vi "Lockin-4461_Multiple Inputs and Outputs_KH_functional_global_waveform_3.vi"(8 "stop":bool) -> ()   [LabVIEW 2013]
uses:
  <vilib>/Analysis/4window.llb/windowTd.ctl
  <vilib>/DAQmx/write.llb/DAQmx Write (Analog 1D Wfm NChan NSamp).vi
  <vilib>/Analysis/baseanly.llb/Mean (DBL).vi
  <vilib>/Analysis/2dsp.llb/Decimate (single shot).vi
  <vilib>/Analysis/2dsp.llb/Decimate (single shot, DBL).vi
  DAQ-Lockin-SubVI/Lock-in Globles Multiple Inputs and Outputs used with FGV.vi
  <vilib>/DAQmx/miscellaneous.llb/DAQmx Fill In Error Info.vi
  <vilib>/Utility/error.llb/Error Cluster From Error Code.vi
  <vilib>/measure/madcrms.llb/Basic Averaged DC-RMS for N Chan.vi
  <vilib>/measure/macond.llb/IIR Filter for N Chan.vi
  <vilib>/measure/maspectr.llb/FFT Power Spectrum and PSD for N Chan.vi
  <vilib>/Analysis/NI_AALBase.lvlib
  <vilib>/measure/NI_MAPro.lvlib
  <vilib>/measure/NI_MABase.lvlib
  <vilib>/Analysis/NI_AALPro.lvlib
panel:
  in  "order":i32=2
  in  "TC (s)":dbl
  out "filter fC (Hz)":dbl
  in  "Input Signals":i16(slide)=2 scale=1.0..20.0
  out "phase log":dbl[](array[numeric])=[0.0, 0.0, 0.0, 0.0, 0.0, 6.661338147750939e-16, 0.0, 1.9984014443252818e-15]
  in  "Tab Control 2":T1(tab)=enum."Lock-in Settings"
  in  "Auto control  max AI rate/ AI block size":bool=TRUE
  in  "AI Buffer Size (S)":i32=10
  in  "AI Block Size":i32=1000
  in  "AI Configuration":T2(array[cluster])=[{"AI.Coupling"=10050, "AI.Max"=10.0, "AI.Min"=-10.0, "Input physical channels"="PXI1Slot2/ai0:1"}, {"AI.Coupling"=10050, "AI.Max"=10.0, "AI.Min"=-10.0, "Input physical channels"="PXI1Slot3/ai0:1"}, {"AI.Coupling"=10050, "AI.Max"=10.0, "AI.Min"=-10.0, "Input physical channels"="PXI1Slot5/ai0:1"}, {"AI.Coupling"=10050, "AI.Max"=10.0, "AI.Min"=-10.0, "Input physical channels"="PXI1Slot6/ai0:1"}] {"AI.Coupling" items=["AC"=10045, "DC"=10050, "GND"=10066]}
  in  "AO Configuration":T3(array[cluster])=[{"Output physical channels"="PXI1Slot2/ao0:1", "AO. Max"=0.1, "AO.Min"=-0.1}, {"Output physical channels"="PXI1Slot3/ao0:1", "AO. Max"=0.25, "AO.Min"=-0.25}, {"Output physical channels"="PXI1Slot5/ao0:1", "AO. Max"=0.1, "AO.Min"=-0.1}, {"Output physical channels"="PXI1Slot6/ao0:1", "AO. Max"=0.1, "AO.Min"=-0.1}]
  in  "OSC Configuration":T4(array[cluster])=[[{"Signal Type"=enum."Sine Wave", "DC"=0.0, "Amplitude"=0.01, "frequency"=13.0, "Phase"=0.0}, {"Signal Type"=enum."Sine Wave", "DC"=0.0, "Amplitude"=0.0, "frequency"=13.0, "Phase"=0.0}], [{"Signal Type"=enum."Sine Wave", "DC"=0.0, "Amplitude"=0.0, "frequency"=13.0, "Phase"=0.0}, {"Signal Type"=enum."Sine Wave", "DC"=0.0, "Amplitude"=0.0, "frequency"=13.0, "Phase"=0.0}], [{"Signal Type"=enum."Sine Wave", "DC"=0.0, "Amplitude"=0.0, "frequency"=13.0, "Phase"=0.0}, {"Signal Type"=enum."Sine Wave", "DC"=0.0, "Amplitude"=0.0, "frequency"=13.0, "Phase"=0.0}], [{"Signal Type"=enum."Sine Wave", "DC"=0.0, "Amplitude"=0.0, "frequency"=13.0, "Phase"=0.0}, {"Signal Type"=enum."Sine Wave", "DC"=0.0, "Amplitude"=0.0, "frequency"=13.0, "Phase"=0.0}]] {"frequency" step=0.001 format="%.3p"; "Amplitude" format="%0.2p"; "DC" min=-0.99 max=0.99 format="%.2p"}
  in  "Phase&Tc":T5(array[cluster])=[{"Phase"=0.0, "Time constant"=0.5, "Set Tc"=FALSE, "Autophase"=FALSE, "Order"=0.0}, {"Phase"=0.0, "Time constant"=0.5, "Set Tc"=FALSE, "Autophase"=FALSE, "Order"=0.0}, {"Phase"=0.0, "Time constant"=0.5, "Set Tc"=FALSE, "Autophase"=FALSE, "Order"=0.0}, {"Phase"=0.0, "Time constant"=0.5, "Set Tc"=FALSE, "Autophase"=FALSE, "Order"=0.0}, {"Phase"=0.0, "Time constant"=0.5, "Set Tc"=FALSE, "Autophase"=FALSE, "Order"=0.0}, {"Phase"=0.0, "Time constant"=0.5, "Set Tc"=FALSE, "Autophase"=FALSE, "Order"=0.0}, {"Phase"=0.0, "Time constant"=0.5, "Set Tc"=FALSE, "Autophase"=FALSE, "Order"=0.0}, {"Phase"=0.0, "Time constant"=0.5, "Set Tc"=FALSE, "Autophase"=FALSE, "Order"=0.0}] {"Phase" min=0.0 max=360.0 scale=0.0..360.0}
  in  "Gain":dbl[](array[numeric])=[50000000.0, 50000000.0, 1.0, 1.0, 1.0, 1.0, 1.0, 1.0]
  in  "frequency":dbl=13.0
  out "max ai rate":i32=13000
  out "elapsed time":dbl=138.0
  in  "zero offset":bool
  in  "measure offset":bool
  in  "sample clock multiple (x*f)":i32=1000
  out "AI Rate":dbl=13000.0 format="%.2f"
  out "Display 2":string="-423.350804      n"
  out "Display 1":string="-104.244723      n"
  in  "Remote":bool
  in  "Display":u16(ring) items=["X and Y", "R and Theta"]
  out "Backlog":u8(slide) scale=0.0..100.0
  out "Sampling information":cluster{"Fs":dbl, "#s":dbl}[](array[cluster])=[{"Fs"=13000.0, "#s"=1000.0}]
  out "AO Task":refnum<k21>[](array[refnum])
  out "AI task":refnum<k21>[](array[refnum])
  in  "Tab Control":T6(tab)=enum."Input signals"
  out "Display X (or R) A":dbl[](graph)=[-6.767704118237299e-07, 1.3679095941982762e-06, -8.292119972514093e-07, 1.6081112063430916e-06, -6.48302849428553e-07, 3.3000787620994813e-07, 2.1826626593165523e-07, -4.843594448984296e-07, 7.025229913353154e-07, -4.940803961923873e-07, 5.735003337473624e-07, -3.4668515755027405e-07, -2.4248283537339965e-07, -1.8363287469697745e-08, -3.4589425846339534e-07, 4.6284358832454705e-07, -2.6962179655822256e-07, -1.429402751088828e-07, 9.446578651191532e-08, -5.710117984178673e-09, -5.29242574030563e-07, -7.215176081254315e-08, 2.677231693663559e-07, -2.9474346178622007e-07, 1.6859037233620488e-07, -2.782624102402718e-07, -1.9986912438858682e-07, -3.269593679273288e-08, -2.486510407656373e-07, 5.548402109992747e-07, 9.996987486709427e-08, -6.0130416412624e-08, 9.415818662231201e-08, -2.1083634639079388e-07, 4.091053197976716e-07, -1.1752425483839359e-08, -6.151119173511262e-08, 4.276364767795889e-07, 5.672540816315234e-09, 1.9631938693768442e-07, 3.881923939998436e-07, 3.693414665428258e-07, 2.2443312885204412e-07, -1.0424472343376792e-07, -3.281356459413585e-06, 2.853877661113482e-06, -1.6173510513608656e-06, 2.900242509974247e-07, 3.0449767746807755e-07, -9.53094648189971e-07, 1.19768766975668e-06, -1.6300022513090843e-06, 1.2633381081086798e-06, -1.2597657763077924e-06, 1.5181775758183967e-06, -3.2698180448977813e-07, 4.534684182323745e-22, 2.954958383906869e-22, 2.935987294164666e-22, 2.9919274066034985e-22, 2.4866884846013956e-11, 1.571439962444634e-06, 3.5981993954562916e-05, 4.595320866342681e-05, -3.163614064440566e-05, 2.2025345770237146e-05, -1.4783690228833628e-05, 9.027427496250188e-06, -4.373865947312203e-06, 1.2061179513411652e-06, 2.321934449801555e-06, -3.096117951559957e-06, 3.818767600136303e-06, -2.724223846911526e-06, 2.777457898492608e-06, -1.6318104191727555e-06, 8.644446773102741e-07, 5.245164233996108e-07, -9.074912983112755e-07, 1.5809479476204886e-06, -1.191807434600212e-06, 1.1136104668741203e-06, -8.918436045180084e-07, 7.666775683008394e-07, 4.0094363870758105e-07, -5.024016863890059e-07, 6.184199345905923e-07, -4.547811927193765e-07, 8.577352486006216e-07, -3.929716458984687e-07, -9.250952352542821e-08, 1.4464495001439634e-07, 2.987012020098487e-07, -8.395621078021276e-09, -5.946540278253675e-08, 5.015724336232653e-07, -2.2845172399208505e-07, 2.9148694268542234e-07, -3.3585825169289965e-08, 1.5255809451280384e-07, -1.6688588171069325e-07, 2.9208673634758535e-07, 2.1867560915340566e-08, -1.817033331852077e-09, 2.0922044023006386e-07, -2.0089195447457524e-07, -1.6047621413178067e-07, 3.62693951906398e-07, -4.219972565448854e-07, 2.644775088575862e-07, 1.6782279517097728e-07, -4.0780410649598406e-07, -1.4202551172988562e-07, 4.1098274242707864e-08, 4.0982393853747056e-07, -1.0954576241181e-08, -2.000666884411931e-07, 3.419460779804609e-07, -5.831329333541703e-07, 1.607889368959098e-07, 4.7485928317065607e-07, -1.0986820397700458e-07, 4.234349182513178e-07, 7.50799000900104e-09, -2.913745535551743e-07, 5.212516629832497e-07, -3.5679666811606247e-07, 7.185358920930657e-07, 2.28551626188166e-07, 2.984900132189184e-07, 5.567614355159372e-07, -2.700163649574881e-08, 4.647757728519345e-09, -7.827331963284188e-09, -3.16290394262067e-07, 2.2708072760302243e-07, 7.739366205819891e-08, -4.86859103219973e-07, 2.473259207485168e-07, -3.41601067670072e-07, 1.6627441476941349e-07, 8.910868327391612e-08, -4.126919161116403e-08, 5.064621322918384e-07, -7.216585649893412e-08, 1.7360798289963554e-07, 1.9894946958931327e-07, -1.029870892195247e-07, 1.479174782511515e-08, -7.761128801091328e-08, -9.710807258322806e-08, 2.244692789108791e-07, -5.009546674149695e-07, 2.4630441386600876e-07, 3.701090240857261e-07, -4.940910423104556e-07, 6.97823655978583e-07, 5.463396637012674e-08, 3.3460509656657584e-07, 1.1628795209397034e-07, -9.983904012316269e-08, 2.1194575699660896e-07, -1.4284598126625291e-07, -1.6581535570295627e-07, 1.9543419229659077e-07, 6.421246147653625e-08, 3.817631543808754e-07, 3.5099411367530134e-07, 9.599061510866204e-08, 5.115460403448378e-07, -3.189544820970916e-07, 2.0371122850583007e-07, 7.139469677112191e-08, -2.6780725397357064e-08, 1.8207931762268008e-07, -3.99163483902508e-08, 3.5667336283414435e-24, 2.977721146793187e-22, 2.9488566597725565e-22, 2.931805455672584e-22, 2.8533874679319433e-11, 4.4171853288673887e-07, 1.1776020155369053e-05, 4.5492863810876877e-05, 2.9323742019926304e-05, -2.1525943992685573e-05, 6.085028499678217e-06, 3.4517457636324723e-06, -7.402821485273008e-06, 8.023515280656284e-06, -5.743846711537538e-06, 3.3274091105157146e-06, -7.62703220096605e-07, -1.0696366449954687e-06, 2.5134804524775262e-06, -2.6343637407641244e-06, 2.5318619928474184e-06, -1.7306766758057638e-06, 1.44992950833644e-06, 1.4483945167047895e-07]
  out "Display Y (or Theta) A":dbl[](graph)=[4.765499299686936e-07, -9.658586916637982e-07, -7.621778309143253e-08, -1.5258147249425879e-07, -2.4990753387284357e-07, 1.3419411932204113e-07, -8.565299692875945e-07, 5.571108791407577e-07, -7.860547079397809e-08, -7.196286228942718e-07, 3.4315278763967647e-07, -6.204384175643328e-07, 1.774316085303007e-07, 1.375503590545208e-07, -9.027207823009459e-07, 4.7108028753992357e-07, -1.4273262355224388e-07, -5.084378639622054e-07, 2.0064639544519283e-07, -6.100241361118937e-07, 3.5508186140312606e-07, 1.6599492404614552e-07, -1.1241242632694126e-06, 3.545737663988187e-07, -1.3680834360003273e-07, -5.671646797482132e-07, 3.003111466009731e-07, -7.790822713575479e-07, 3.293880422749827e-07, 3.28274379240407e-08, -1.0651740914596076e-06, 4.2770794764999845e-07, -5.104224380786051e-07, -2.472151922016114e-07, 1.9800282516829894e-07, -7.284254119168647e-07, 5.863115303219669e-07, -2.81773970579004e-07, -7.156335675351997e-07, 2.3981773570157667e-07, -3.978801443495009e-07, 3.035512690481674e-07, -1.7158995838277135e-07, -4.233508035480193e-07, -8.088850970477616e-07, 6.737027936126898e-07, -1.759072178658265e-07, -6.972834404887968e-07, 1.272488135816818e-06, -1.2086621076536852e-06, 4.69525474705048e-07, -4.919175010780031e-08, -3.50864282590232e-07, 6.020350472256037e-07, -9.484640076506137e-07, -6.830224693863262e-08, 1.0170935534147539e-22, -8.29623972830081e-22, -8.014563293027786e-22, -8.094000243152346e-22, 1.3353078985706605e-11, 1.6373548472325611e-07, 1.4866311767580978e-06, -2.707411790797605e-06, 6.830995141435044e-07, -3.8763934216822793e-07, -3.894235373830128e-07, -9.303274404957174e-08, -1.5541472171160917e-07, -1.0548850159824638e-06, 1.301686262269789e-06, -1.9557074574821375e-06, 9.368644690210887e-07, -5.392324932206546e-07, -1.0317815283114626e-06, 9.503284335604831e-07, -1.1138402195810916e-06, -8.612001299094237e-08, 3.392287632745269e-07, -9.880574731396456e-07, 6.176942647460194e-07, -5.670403477561947e-07, -7.529082791811021e-08, 3.797538713075729e-07, -6.875418705429333e-07, 3.774689030428864e-08, 4.010310610815791e-07, -5.552428738314573e-07, 3.8499536868861883e-07, -6.445873434134007e-07, -3.326615731244241e-07, 4.502182873700019e-07, -7.750874192225206e-07, 4.117923202917222e-07, -6.431352998299419e-07, 3.5044644716276235e-07, -1.4225277208615523e-07, -6.876478797176894e-07, 5.399420578514256e-07, -4.5606838526251626e-07, -1.2810883746936567e-07, 7.507205080273586e-07, -1.4012460201934012e-06, 3.6687827494239255e-07, -2.4916075902104696e-07, -6.048091008906423e-07, 6.617540494081048e-07, -1.017139965154715e-06, 6.302573641557335e-07, 4.555496901851896e-07, -1.3339391648309178e-06, 6.715666266662573e-07, -3.8798990954152797e-07, -3.6012440675569084e-07, 5.414910168700109e-07, -1.3243576755919245e-06, 5.902559482413635e-07, -7.542190392147796e-08, -1.0785352133753382e-06, 9.869413956855774e-07, -9.442478036537707e-07, -4.8555902344221593e-08, 5.874045024703844e-07, -1.1585692990263365e-06, 1.3486079750496373e-06, -5.071584526584705e-07, -5.100916917445276e-07, 6.330937674492109e-07, -1.235592399497452e-06, 9.223862720486185e-07, 6.04251856246877e-08, -1.2764854943402043e-06, 8.83547168218078e-07, -9.047288617993288e-07, 2.0116909352114474e-07, 5.358138396845644e-07, -1.3168565866224215e-06, 4.095307061714363e-07, -6.27867381040266e-07, -4.472555022141913e-07, 8.124683056348434e-07, -6.96815296189946e-07, -1.3075261738966236e-07, -2.448175089906454e-07, -3.31091978464826e-07, 4.938406467055916e-07, -1.0121928097926847e-06, 2.6683471402237015e-07, -3.854622779756573e-07, -6.116229848120615e-07, 7.413846592203119e-07, -3.878576789341664e-07, -4.803212369821987e-09, -1.512740254582647e-07, -9.37733298786493e-07, 3.083451264193004e-07, -7.278473080315107e-07, -2.1621978373244913e-07, 1.1649243053043013e-06, -1.5574296555740364e-06, 2.0216029416288657e-07, -1.738290377715283e-08, -8.124252331847678e-07, 8.556517228357048e-07, -1.1895268912765046e-06, -1.6299284686030149e-07, 5.025591222770188e-07, -1.256876728303257e-06, 4.966801881381768e-07, -2.653578297740131e-07, -7.841925208481243e-07, 6.961355949365849e-07, -1.3545884441334733e-06, 1.8978106285789698e-07, -3.1292466455277164e-07, -1.116079741754174e-06, 6.606025379921262e-24, -7.987352443116322e-22, -8.305769155450611e-22, -8.014315043874178e-22, 1.528632786785048e-11, 5.851716352372578e-08, 7.012774926585611e-07, 7.260202605191567e-07, -1.8385722657507987e-06, -7.48491270371179e-07, 1.078630704871155e-06, -5.895807456908318e-07, 1.4658536078852006e-07, 1.0975439156015532e-07, -4.165723785464372e-07, -6.413089995227893e-08, 2.3302809137460278e-07, -4.5082625792713e-08, 1.8812524970362413e-07, 1.2661990176118822e-08, -9.607065782256097e-07, 4.267709983481109e-07, -7.948677906464168e-08, -2.6388811975329723e-07]
  out "Waveform Graph":waveform(dbl)[](graph)
  in  "decimating factor":i32=1
  in  "simulate?":bool
  in  "pt by pt?":bool
  out "Waveform Graph 2":cluster{"f0":dbl, "df":dbl, "magnitude":dbl[]}[](graph)
  in  "window":T7=1 items=["Rectangle"=0, "Hanning"=1, "Hamming"=2, "Blackman-Harris"=3, "Exact Blackman"=4, "Blackman"=5, "Flat Top"=6, "4 Term B-Harris "=7, "7 Term B-Harris"=8, "Low Sidelobe"=9, "Blackman Nuttall"=11, "Triangle"=30, "Bartlett-Hanning"=31, "Bohman"=32, "Parzen"=33, "Welch"=34, "Kaiser"=60, "Dolph-Chebyshev"=61, "Gaussian"=62]
  in  "averaging parameters":T8={"averaging mode"=enum."No averaging", "weighting mode"=enum."Exponential", "number of averages"=10} {"number of averages" min=1}
  in  "dB On (F)":bool
  out "Results (X, Y, R, Theta)":dbl[][](array[numeric])=[[-8.990938951699043e-08, -5.496874633933286e-07, 5.569919260950825e-07, -99.28930194172699], [-1.0424472343376792e-07, -4.233508035480193e-07, 4.3599640506377615e-07, -103.83315475232594], [-8.663279130692378e-08, -2.555950511771059e-07, 2.6987788111636043e-07, -108.72385784210852], [-3.572835649086049e-08, -7.56786271488616e-08, 8.368853006639814e-08, -115.2722910768039], [4.431812686724637e-08, 8.517364090161592e-08, 9.601377751895176e-08, 62.51083208252897], [1.4523643643592666e-07, 1.9896598237318188e-07, 2.4633530930488284e-07, 53.87219602328508]] format="%#_6p"
  out "Measure?":u16[](array[numeric])
  in  "Cluster (unused right now)":T9={"Amplitude"=[0.001, 2e-08, 0.001, 0.001, 0.001, 2e-08], "DC"=[0.001, 2e-08, 0.001, 0.001, 0.001, 2e-08], "phase"=[0.001, 2e-08, 0.001, 0.001, 0.001, 2e-08], "Array"=[]}
  out "offsets":dbl[](array[numeric])
  # "*****Customized for 4461 + 4462 cards; functional globals*****"
  # "Real time Adjustable Values"
  # "WAVEFORM 2"
  # "Configurations"
  # "should this be x multiple\nof the frequency?"
  # "The top array index selects which card you are setting the outputs for,and the second index selects which output chanel on that card.\n\nFor Phase&Tc, you must have an array element initialized for each input signal."
  # "Features:\n1, Any number of input and output channels\n2, Each AO outputs an DC+AC signal, DC for sample biasing and AC for OSC. These values can be adjusted in real time.\n3, Synchronous filtering\n\nInstructions:\n1, Array index of AI configuration and AO configuration refers to task.\n2, Array index in Amplifier Settings, Phase$&Tc control , and gains correlates to channel number.\n3, Each 4461 board can have 2 lock-in channels. Syntax for 2 channles, e.g. PXI1Slot2/ai0:1. If you want to use just one, then PXI1Slot2/ai0.\n4, Parameters (especially DC value for sample biasing) can be remotely controlled by clicking \"local\"and \"remote\" button. In real experiments, put golable values (can be found in Lock-in globles.vi) in your VI to control the lock-in and read out.\n5, choose OSC frequencies to be multiple of \nAI Rate/AI Block SIze to have best performance.\n\n-Guanglei 06/23/2011\n\nUpdate:\n1. Allows any number of lockin amplifiers and AO tasks.\n2. Delete the channels from any AI/AO Configuration elements you do not want to use.\n3. Rows (first index) of the OSC Configuration correspond to different AO tasks, while columns (second index) correspond to AO channels in that task. All channels in a given element of the AO Configuration array will go into a single task.\n4. The same number of output channels must go in each AO task.\n5. Make sure a Phase&Tc element and an Amplifier Settings element is set for each AI channel.\n-Joe 12/3/2013"
  # "signal\n*sine\n*cosine\n*2\n*2\nLP filter\nLP filter"
  # "hide stuff here in this tab"
  # "multiple of frequency??"
  # "this is \"time constant\""
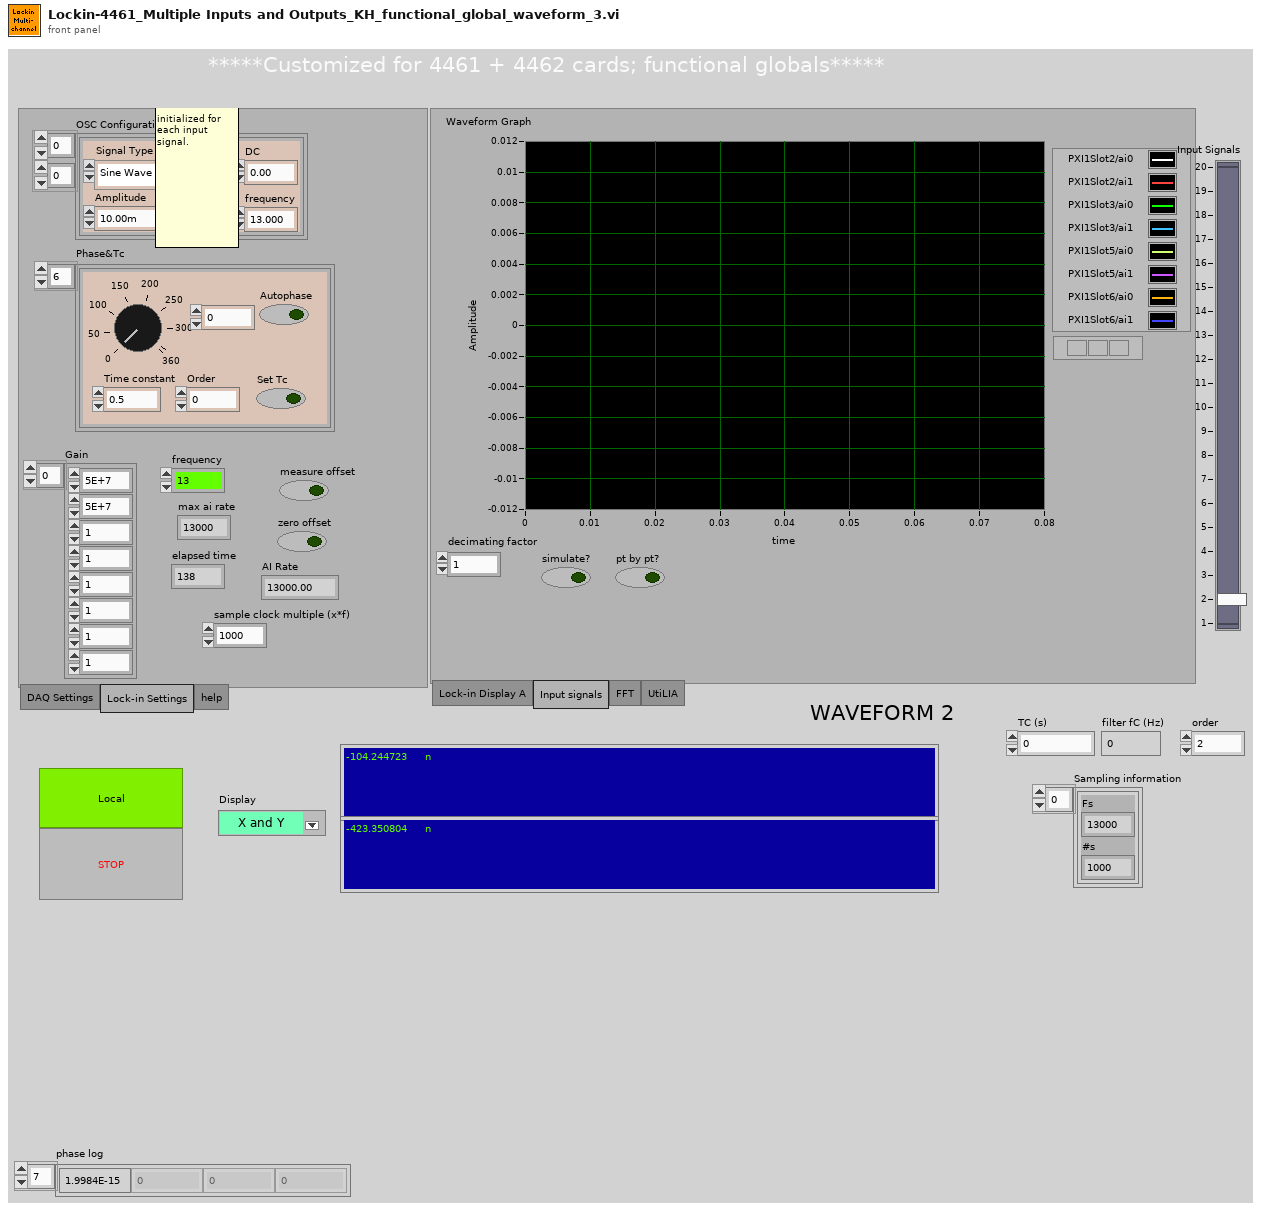
[diagram p1: front panel]
types:
  T1 = enum32{"DAQ Settings", "Lock-in Settings", "help"}
  T2 = cluster{"AI.Coupling":i32, "AI.Max":dbl, "AI.Min":dbl, "Input physical channels":tag}[]
  T3 = cluster{"Output physical channels":tag, "AO. Max":dbl, "AO.Min":dbl}[]
  T4 = cluster{"Signal Type":enum16{"Sine Wave", "Triangle Wave", "Square Wave", "Sawtooth Wave"}, "DC":dbl, "Amplitude":dbl, "frequency":dbl, "Phase":dbl}[][]
  T5 = cluster{"Phase":dbl, "Time constant":dbl, "Set Tc":bool, "Autophase":bool, "Order":dbl}[]
  T6 = enum32{"Lock-in Display A", "Input signals", "FFT", "UtiLIA"}
  T7 = typedef "NI_AALPro.lvlib/windowTd.ctl" = u32
  T8 = cluster{"averaging mode":enum16{"No averaging", "Vector averaging", "RMS averaging", "Peak hold"}, "weighting mode":enum16{"Linear", "Exponential"}, "number of averages":u32}
  T9 = cluster{"Amplitude":dbl[], "DC":dbl[], "phase":dbl[], "Array":enum16{"Sine Wave", "Triangle Wave", "Square Wave", "Sawtooth Wave"}[]}
  T10 = cluster{"Topology":enum16{"Off", "Butterworth", "Chebyshev", "Inverse Chebyshev", "Elliptic", "Bessel"}, "Type":enum16{"Lowpass", "Highpass", "Bandpass", "Bandstop"}, "Order":i32, "Lower Fc":dbl, "Upper Fc":dbl, "PB Ripple":dbl, "SB Attenuation":dbl}
  T11 = cluster{"Signal Type":enum16{"Sine Wave", "Triangle Wave", "Square Wave", "Sawtooth Wave"}, "DC":dbl, "Amplitude":dbl, "frequency":dbl, "Phase":dbl}
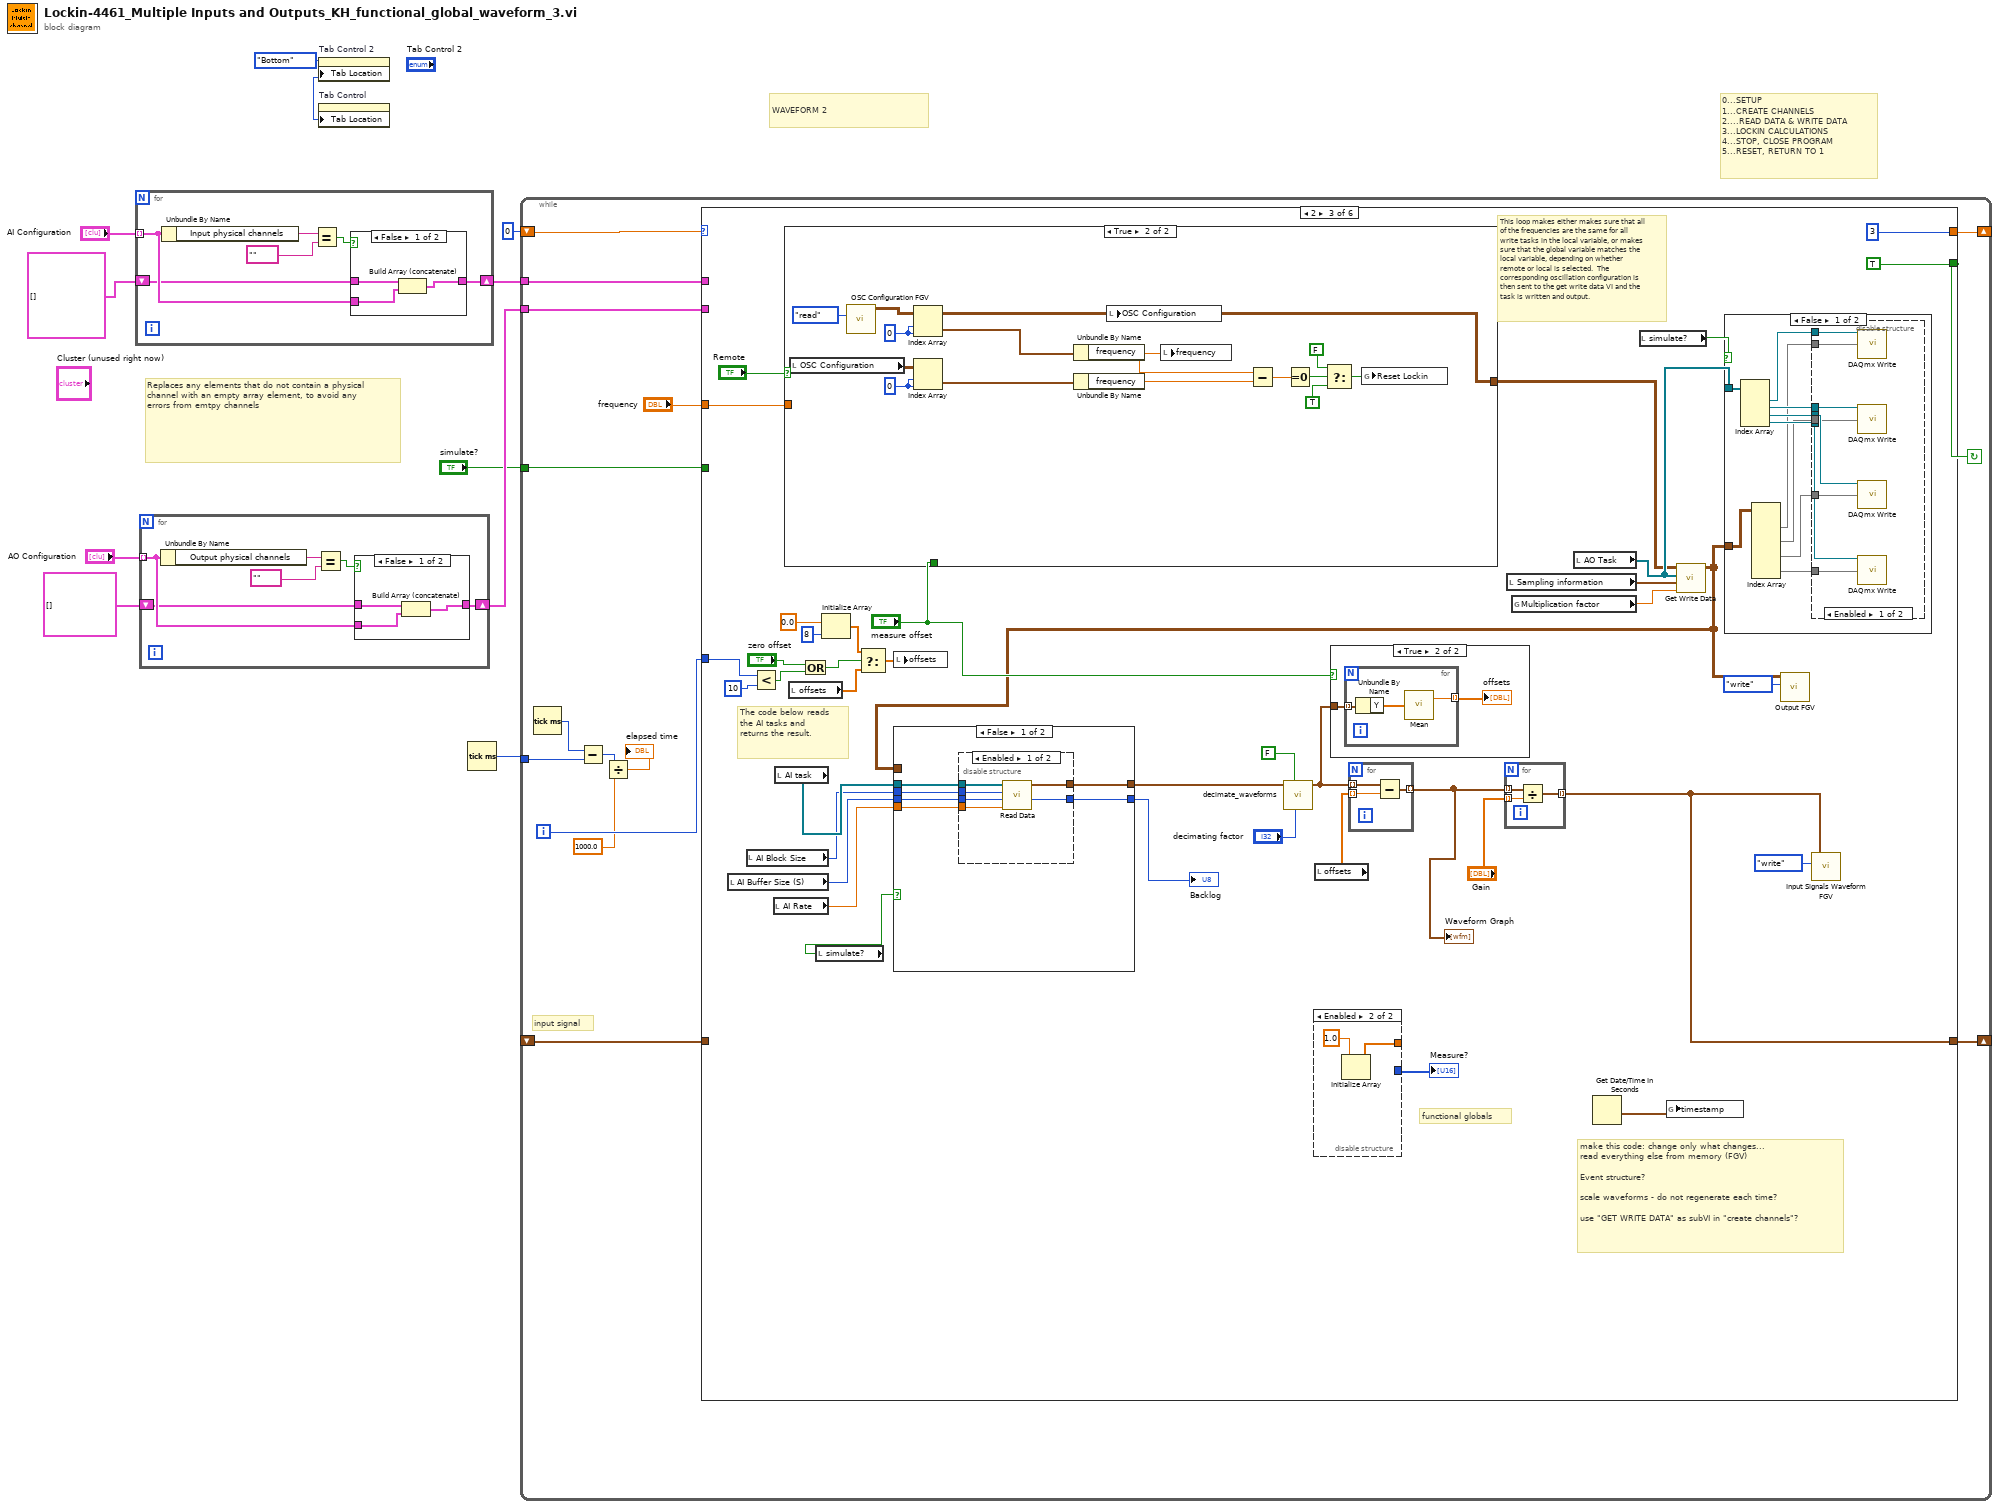
[diagram p0: block diagram]
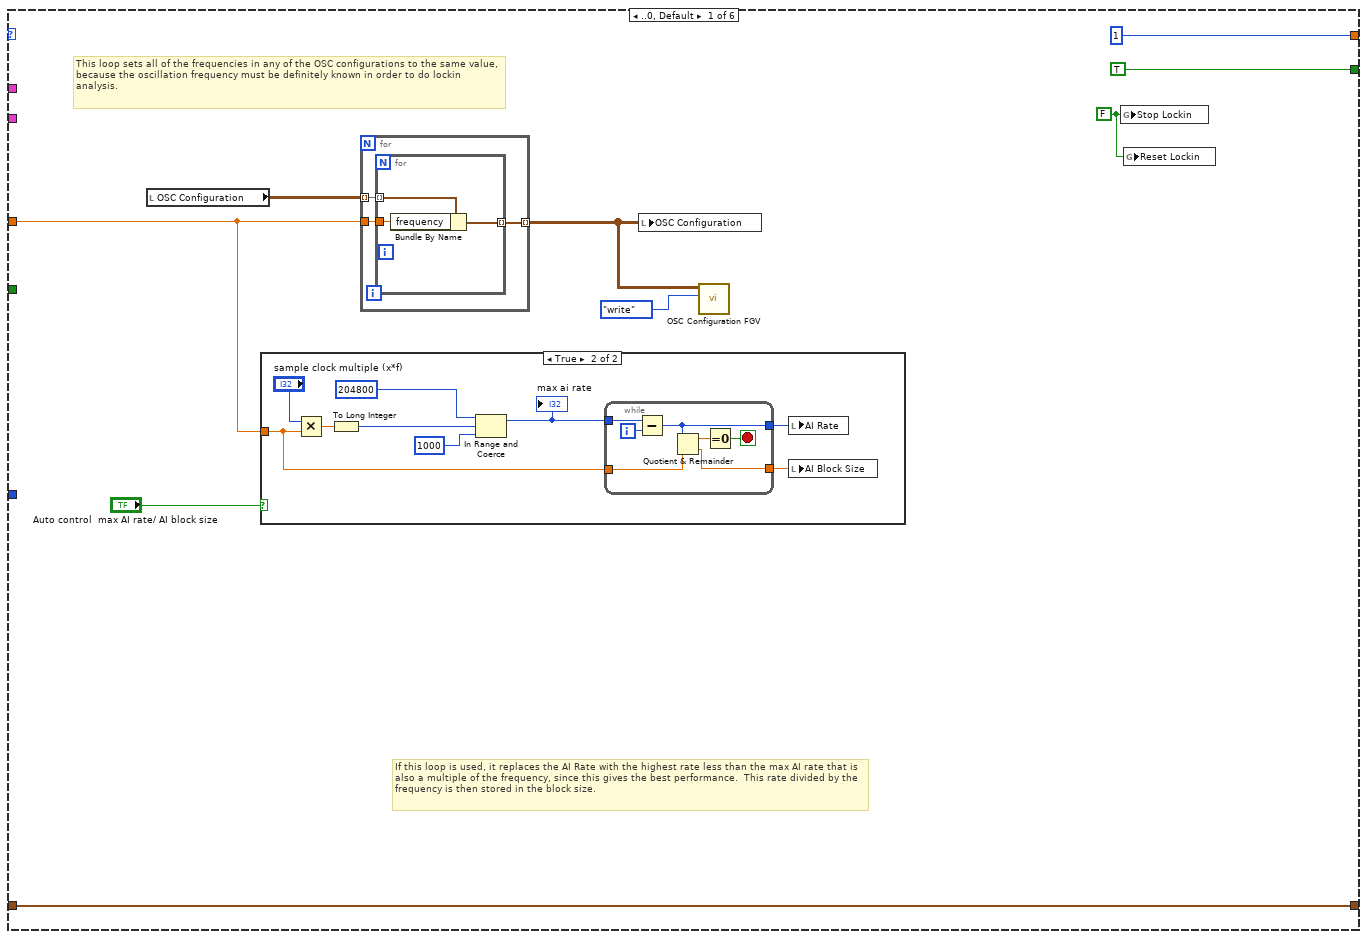
[diagram p4: hidden frame]
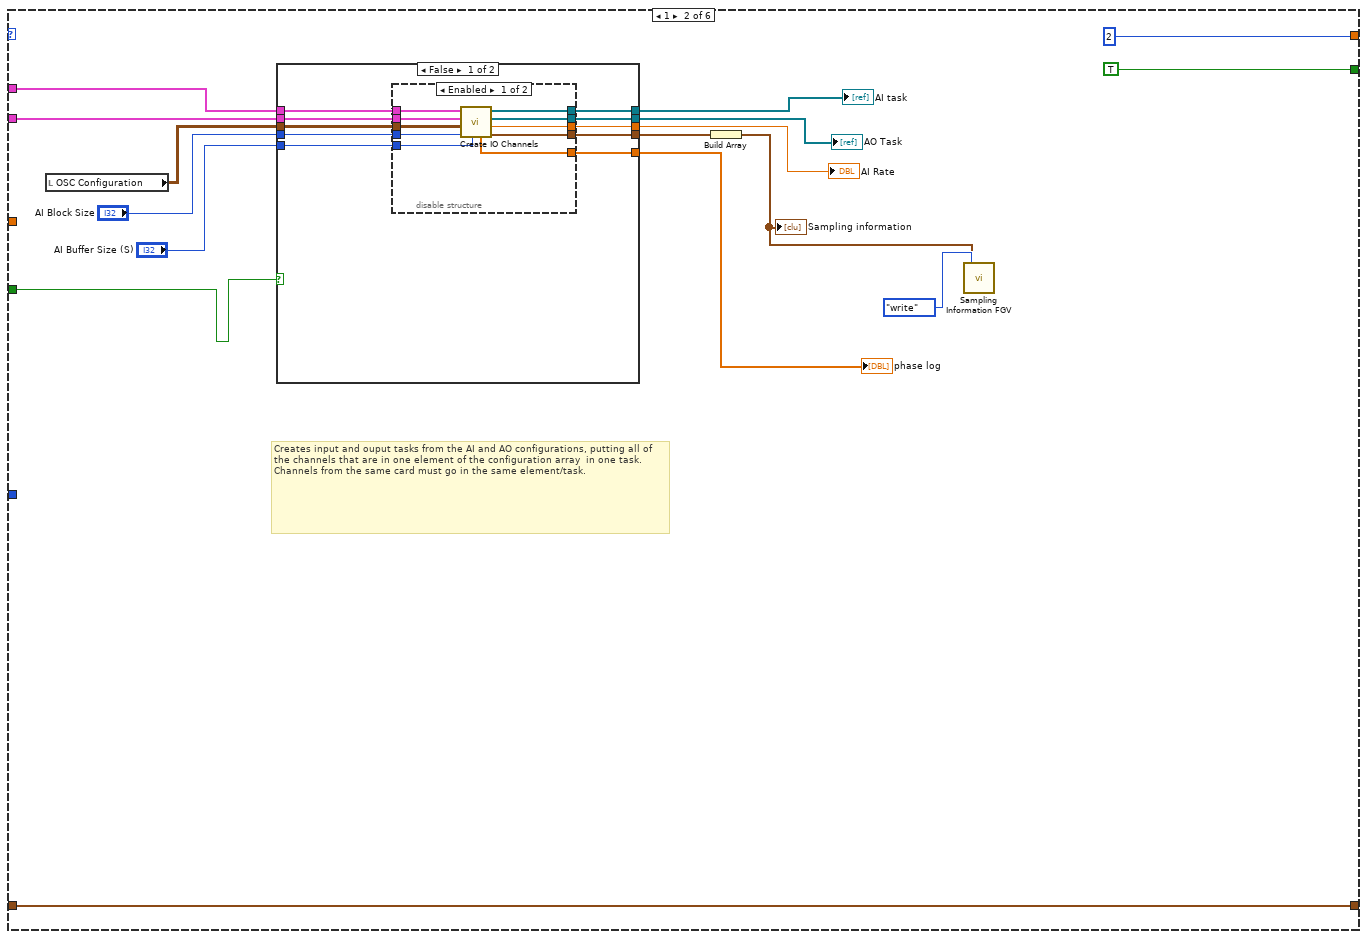
[diagram p6: hidden frame]
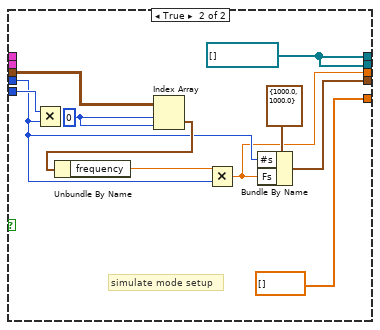
[diagram p8: hidden frame]
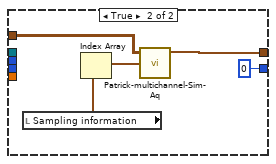
[diagram p12: hidden frame]
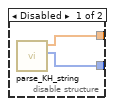
[diagram p14: hidden frame]
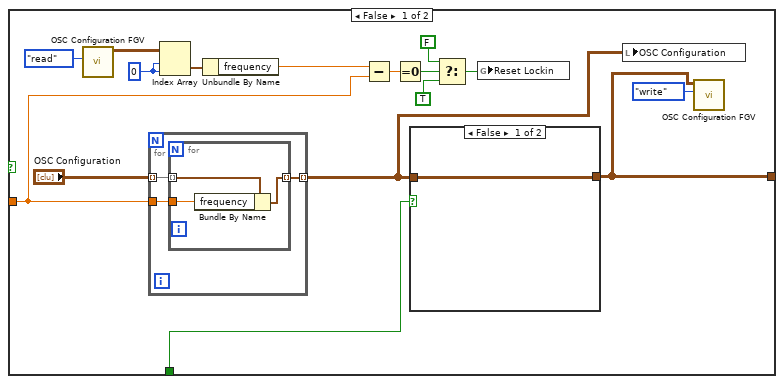
[diagram p15: hidden frame]
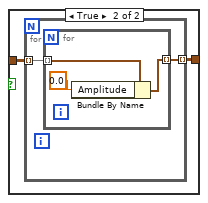
[diagram p16: hidden frame]
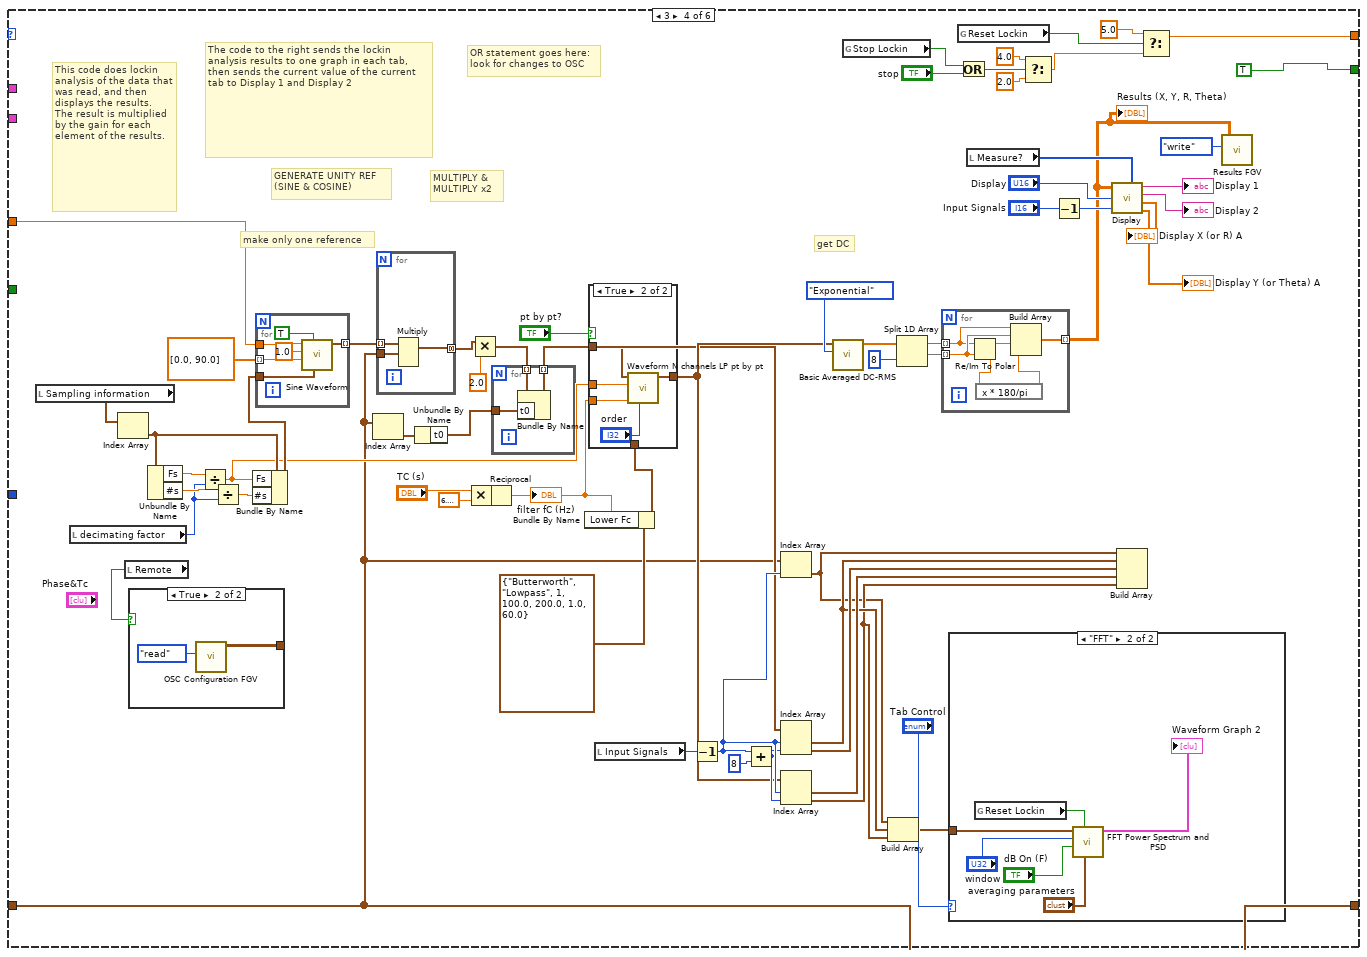
[diagram p17: hidden frame]
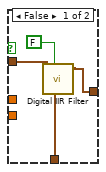
[diagram p18: hidden frame]
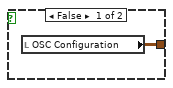
[diagram p20: hidden frame]
diagram:
  w5 = enum32{"Top", "Bottom", "Left", "Right"}."Bottom" ("Tab Location")
  # "0...SETUP\n1...CREATE CHANNELS\n2....READ DATA & WRITE DATA\n3...LOCKIN CALCULATIONS\n4...STOP, CLOSE PROGRAM\n5...RESET, RETURN TO 1"
  # "WAVEFORM 2"
  # "Replaces any elements that do not contain a physical channel with an empty array element, to avoid any errors from emtpy channels"
  n1 = for {
    tunnel: "AI Configuration" -> [w13] mode=indexing
    shift-right: [w11] -> w10
    shift-left: T2 [] ("AI Configuration") -> [w12]
    n2 = Unbundle By Name(w13) -> ("Input physical channels"=w15:tag)
    n3 = Equal?(x=w15, y=tag "" ("Empty physical channels")) -> (x = y?=w16:bool)
    n4 = case shown="False" w16 {
      tunnel: w13 -> [w18 _]
      tunnel: w12 -> [w19 w20]
      tunnel: [w17 w20] -> w11
      frame False {
        n5 = Build Array (concatenate)(w19, w18) -> (w17:T2)
      }
      frame True {
      }
    }
  }
  n6 = for {
    tunnel: "AO Configuration" -> [w23] mode=indexing
    shift-right: [w21] -> w3
    shift-left: T3 [] ("AO Configuration 2") -> [w22]
    n7 = Unbundle By Name(w23) -> ("Output physical channels"=w25:tag)
    n8 = Equal?(x=w25, y=tag "" ("Empty physical channels")) -> (x = y?=w26:bool)
    n9 = case shown="False" w26 {
      tunnel: w23 -> [w28 _]
      tunnel: w22 -> [w29 w30]
      tunnel: [w27 w30] -> w21
      frame False {
        n10 = Build Array (concatenate)(w29, w28) -> (w27:T3)
      }
      frame True {
      }
    }
  }
  n11 = property on="Tab Control 2" class="TabCtl (strict)"("Tab Location"=w5) -> ()  [unwired: 2 in, 2 out]
  n12 = property on="Tab Control" class="TabCtl (strict)"("Tab Location"=w5) -> ()  [unwired: 2 in, 2 out]
  n13 = Tick Count (ms)() -> (millisecond timer value=w2:u32)
  n14 = while {
    shift-right: [w45] -> _
    shift-left: 0 -> [w44]
    tunnel: w10 -> [w43]
    tunnel: w3 -> [w41]
    shift-right: [w40] -> _
    shift-left: _ -> [w39]
    tunnel: w2 -> [w35]
    tunnel: "simulate?" -> [w31]
    i -> [w38]
    stop <- w42 continue-if-true
    # "input signal"
    n15 = Tick Count (ms)() -> (millisecond timer value=w36:u32)
    n16 = Subtract(x=w36, y=w35) -> (x-y=w34:u32)
    n17 = Divide(x=w34, y=1000.0) -> (x/y=→"elapsed time":dbl)
    n18 = case shown="2" w44 {
      selector: w44 -> [_ _ _ _ w358 _]
      tunnel: [1 2 3 w311 w358 0.0 ("f")] -> w45
      tunnel: w43 -> [_ w89 _ _ _ _]
      tunnel: [TRUE TRUE TRUE TRUE FALSE TRUE] -> w42
      tunnel: w41 -> [_ w88 _ _ _ _]
      tunnel: [w47 w83 w125 w257 w357 w387] -> w40
      tunnel: w39 -> [w47 w83 _ w257 w357 w387]
      tunnel: w38 -> [_ _ w149 _ _ _]
      tunnel: "frequency" -> [w46 _ w151 w284 _ _]
      tunnel: w31 -> [_ w77 _ _ _ _]
      frame ..0, Default {
        w53 = FALSE ("Stop Lockin")
        # "If this loop is used, it replaces the AI Rate with the highest rate less than the max AI rate that is also a multiple of the frequency, since this gives the best performance.  This rate divided by the frequency is then stored in the block size."
        # "This loop sets all of the frequencies in any of the OSC configurations to the same value, because the oscillation frequency must be definitely known in order to do lockin analysis."
        n19 = local read "OSC Configuration"() -> (w50:T4)
        n20 = case shown="True" "Auto control  max AI rate/ AI block size" {
          tunnel: w46 -> [_ w61]
          frame False {
          }
          frame True {
            n21 = Multiply(x="sample clock multiple (x*f)", y=w61) -> (x*y=w67:dbl)
            n22 = To Long Integer(number=w67) -> (32bit integer=w65:i32)
            n23 = In Range and Coerce(upper limit=204800, x=w65, lower limit=1000) -> (coerced(x)=w62:i32)  [unwired: 1 out]
            "max ai rate" <- w62
            n24 = while {
              tunnel: w62 -> [w76]
              tunnel: [w74] -> w69
              tunnel: [w72] -> w68
              tunnel: w61 -> [w73]
              i -> [w75]
              stop <- w70 stop-if-true
              n25 = Subtract(x=w76, y=w75) -> (x-y=w72:i32)
              n26 = Quotient & Remainder(x=w72, y=w73) -> (x-y*floor(x/y)=w71:dbl, floor(x/y)=w74:dbl)
              n27 = Equal To 0?(x=w71) -> (x = 0?=w70:bool)
            }
            n28 = local write "AI Rate"(w68) -> ()
            n29 = local write "AI Block Size"(w69) -> ()
          }
        }
        n30 = for {
          tunnel: w50 -> [w57] mode=indexing
          tunnel: [w56] -> w49 mode=indexing
          tunnel: w46 -> [w55]
          n31 = for {
            tunnel: w57 -> [w60] mode=indexing
            tunnel: [w59] -> w56 mode=indexing
            tunnel: w55 -> [w58]
            n32 = Bundle By Name(cluster=w60, "frequency"=w58) -> (w59:T11)
          }
        }
        n33 = local write "OSC Configuration"(w49) -> ()
        n34 = call "OSC Configuration FGV.vi"("Function"=enum16{"write", "read"}."write", "OSC Configuration"=w49) -> ()  [unwired: 4 in, 2 out]
        n35 = global write "Lock-in Globles Multiple Inputs and Outputs used with FGV.vi" "Stop Lockin"(w53) -> ()
        n36 = global write "Lock-in Globles Multiple Inputs and Outputs used with FGV.vi" "Reset Lockin"(w53) -> ()
      }
      frame 1 {
        # "Creates input and ouput tasks from the AI and AO configurations, putting all of the channels that are in one element of the configuration array  in one task.  Channels from the same card must go in the same element/task."
        n37 = local read "OSC Configuration"() -> (w90:T4)
        n38 = case shown="False" w77 {
          tunnel: w90 -> [w102 w121]
          tunnel: w89 -> [w101 _]
          tunnel: w88 -> [w100 _]
          tunnel: [w99 w120] -> w87
          tunnel: [w98 w114] -> w86
          tunnel: "AI Block Size" -> [w97 w117]
          tunnel: [w96 w116] -> w84
          tunnel: [w95 w120] -> w81
          tunnel: "AI Buffer Size (S)" -> [w94 w119]
          tunnel: [w93 dbl[] [] ("phase log")] -> w78
          frame False {
            n39 = disable-structure shown="Enabled" {
              disable-tunnel: w102 -> [w112 _]
              disable-tunnel: w101 -> [w111 _]
              disable-tunnel: w100 -> [w110 _]
              disable-tunnel: [w109 _] -> w99
              disable-tunnel: [w108 _] -> w98
              disable-tunnel: w97 -> [w107 _]
              disable-tunnel: [w106 _] -> w96
              disable-tunnel: [w105 _] -> w95
              disable-tunnel: w94 -> [w104 _]
              disable-tunnel: [w103 _] -> w93
              frame Enabled {
                n40 = call "Create IO Channels.vi"("AI Buffer Size (s)"=w104, "AI Block Size"=w107, "OSC Configuration"=w112, "AO Configuration"=w110, "AI Configuration"=w111) -> ("sampling info"=w106:cluster{"Fs":dbl, "#s":dbl}, "AI Rate"=w108:dbl, "AO Task"=w105:refnum<k21>[], "AI task"=w109:refnum<k21>[], "phase log"=w103:dbl[])  [unwired: 1 in, 1 out]
              }
              frame Disabled {
              }
            }
          }
          frame True {
            w120 = refnum<k21>[] [] ("AI task")
            w122 = 0 ("index (row)")
            # "simulate mode setup"
            n41 = Multiply(x=w119, y=w117) -> ()  [unwired: 1 out]
            n42 = Index Array(array=w121, index (row)=w122, index (col)=w122) -> (element=w118:T11)
            n43 = Unbundle By Name(w118) -> ("frequency"=w123:dbl)
            n44 = Multiply(x=w123, y=w117) -> (x*y=w114:dbl)
            n45 = Bundle By Name(cluster=cluster{"Fs":dbl, "#s":dbl} {"Fs"=1000.0, "#s"=1000.0} ("sampling info"), "#s"=w117, "Fs"=w114) -> (w116:cluster{"Fs":dbl, "#s":dbl})
          }
        }
        "AO Task" <- w81
        "AI Rate" <- w86
        "AI task" <- w87
        "phase log" <- w78
        n46 = Build Array(w84) -> (w80:cluster{"Fs":dbl, "#s":dbl}[])
        "Sampling information" <- w80
        n47 = call "Sampling Information FGV.vi"("Function"=enum16{"write", "read"}."write", "Sampling information"=w80) -> ()  [unwired: 4 in, 2 out]
      }
      frame 2 {
        # "make this code: change only what changes...\nread everything else from memory (FGV)\n\nEvent structure?\n\nscale waveforms - do not regenerate each time?\n\nuse \"GET WRITE DATA\" as subVI in \"create channels\"?"
        # "functional globals"
        # "The code below reads the AI tasks and returns the result."
        # "This loop makes either makes sure that all of the frequencies are the same for all write tasks in the local variable, or makes sure that the global variable matches the local variable, depending on whether remote or local is selected.  The corresponding oscillation configuration is then sent to the get write data VI and the task is written and output."
        n48 = local read "AI Buffer Size (S)"() -> (w154:i32)
        n49 = local read "AI Block Size"() -> (w155:i32)
        n50 = Less?(x=w149, y=10) -> (x < y?=w142:bool)
        n51 = local read "AI Rate"() -> (w153:dbl)
        n52 = local read "AI task"() -> (w156:refnum<k21>[])
        n53 = case shown="True" "Remote" {
          tunnel: [w213 w243] -> w135
          tunnel: w151 -> [w216 _]
          tunnel: "measure offset" -> [w215 _]
          frame False {
            w225 = 0 ("index")
            n54 = call "OSC Configuration FGV.vi"("Function"=enum16{"write", "read"}."read") -> ("OSC Configuration"=w219:T4)  [unwired: 5 in, 1 out]
            n55 = for {
              tunnel: w216 -> [w239]
              tunnel: "OSC Configuration" -> [w238] mode=indexing
              tunnel: [w237] -> w214 mode=indexing
              n56 = for {
                tunnel: w238 -> [w242] mode=indexing
                tunnel: w239 -> [w241]
                tunnel: [w240] -> w237 mode=indexing
                n57 = Bundle By Name(cluster=w242, "frequency"=w241) -> (w240:T11)
              }
            }
            n58 = Index Array(array=w219, index (row)=w225, index (col)=w225) -> (element=w224:T11)
            n59 = Unbundle By Name(w224) -> ("frequency"=w218:dbl)
            n60 = Subtract(x=w218, y=w216) -> (x-y=w217:dbl)
            n61 = Equal To 0?(x=w217) -> (x = 0?=w223:bool)
            n62 = case shown="False" w215 {
              tunnel: w214 -> [w229 w231]
              tunnel: [w229 w230] -> w213
              frame False {
              }
              frame True {
                n63 = for {
                  tunnel: w231 -> [w233] mode=indexing
                  tunnel: [w232] -> w230 mode=indexing
                  n64 = for {
                    tunnel: w233 -> [w236] mode=indexing
                    tunnel: [w235] -> w232 mode=indexing
                    n65 = Bundle By Name(cluster=w236, "Amplitude"=0.0) -> (w235:T11)
                  }
                }
              }
            }
            n66 = Select(t=FALSE ("Reset Lockin"), s=w223, f=TRUE ("Reset Lockin")) -> (s? t:f=w220:bool)
            n67 = global write "Lock-in Globles Multiple Inputs and Outputs used with FGV.vi" "Reset Lockin"(w220) -> ()
            n68 = local write "OSC Configuration"(w214) -> ()
            n69 = call "OSC Configuration FGV.vi"("Function"=enum16{"write", "read"}."write", "OSC Configuration"=w213) -> ()  [unwired: 4 in, 2 out]
          }
          frame True {
            w253 = 0 ("index")
            w255 = 0 ("index")
            n70 = local read "OSC Configuration"() -> (w245:T4)
            n71 = call "OSC Configuration FGV.vi"("Function"=enum16{"write", "read"}."read") -> ("OSC Configuration"=w243:T4)  [unwired: 5 in, 1 out]
            n72 = Index Array(array=w243, index (row)=w255, index (col)=w255) -> (element=w256:T11)
            n73 = Index Array(array=w245, index (row)=w253, index (col)=w253) -> (element=w252:T11)
            n74 = Unbundle By Name(w256) -> ("frequency"=w244:dbl)
            n75 = Unbundle By Name(w252) -> ("frequency"=w250:dbl)
            n76 = local write "OSC Configuration"(w243) -> ()
            n77 = local write "frequency"(w244) -> ()
            n78 = Subtract(x=w244, y=w250) -> (x-y=w251:dbl)
            n79 = Equal To 0?(x=w251) -> (x = 0?=w249:bool)
            n80 = Select(t=FALSE ("Reset Lockin"), s=w249, f=TRUE ("Reset Lockin")) -> (s? t:f=w246:bool)
            n81 = global write "Lock-in Globles Multiple Inputs and Outputs used with FGV.vi" "Reset Lockin"(w246) -> ()
          }
        }
        n82 = local read "offsets"() -> (w148:dbl[])
        n83 = Or(x="zero offset", y=w142) -> (x .or. y?=w141:bool)
        n84 = local read "simulate?"() -> (w129:bool)
        n85 = Initialize Array(0.0, 8 ("dimension size")) -> (w145:dbl[])
        n86 = Select(t=w145, s=w141, f=w148) -> (s? t:f=w147:dbl[])
        n87 = local write "offsets"(w147) -> ()
        n88 = disable-structure shown="Enabled" {
          disable-tunnel: [w210 w211] -> _
          disable-tunnel: [w209 _] -> w150
          frame Disabled {
            n89 = call "parse_KH_string.vi"() -> ("Measurement type"=w209:i32[], "Gain"=w210:dbl[])  [unwired: 10 in]
          }
          frame Enabled {
            n90 = Initialize Array(1.0) -> (w211:dbl[])  [unwired: 1 in]
          }
        }
        "Measure?" <- w150
        n91 = local read "offsets"() -> (w140:dbl[])
        n92 = local read "Sampling information"() -> (w158:cluster{"Fs":dbl, "#s":dbl}[])
        n93 = global read "Lock-in Globles Multiple Inputs and Outputs used with FGV.vi" "Multiplication factor"() -> (w157:dbl)
        n94 = local read "AO Task"() -> (w136:refnum<k21>[])
        n95 = Get Date/Time In Seconds() -> (seconds since 1Jan1904=w159:timestamp)
        n96 = local read "simulate?"() -> (w128:bool)
        n97 = global write "Lock-in Globles Multiple Inputs and Outputs used with FGV.vi" "timestamp"(w159) -> ()
        n98 = call "Get Write Data.vi"("Multiplication Factor"=w157, "Sampling information 2"=w158, "AO Task"=w136, "OSC Configuration"=w135) -> ("Data"=w127:waveform(dbl)[][])  [unwired: 7 in]
        n99 = case shown="False" w129 {
          tunnel: w156 -> [w186 _]
          tunnel: w155 -> [w185 _]
          tunnel: w154 -> [w184 _]
          tunnel: w153 -> [w183 _]
          tunnel: [w182 u8 0 ("Backlog")] -> w126
          tunnel: [w181 w195] -> w132
          tunnel: w127 -> [_ w193]
          frame False {
            n100 = disable-structure shown="Enabled" {
              disable-tunnel: w186 -> [w192 _]
              disable-tunnel: w185 -> [w191 _]
              disable-tunnel: w184 -> [w190 _]
              disable-tunnel: w183 -> [w189 _]
              disable-tunnel: [w188 _] -> w182
              disable-tunnel: [w187 _] -> w181
              frame Enabled {
                n101 = call "Read Data.vi"("AI Rate"=w189, "AI Buffer Size (s)"=w190, "AI Block Size"=w191, "AI task"=w192) -> ("Backlog"=w188:u8, "Input Signals"=w187:waveform(dbl)[])  [unwired: 5 in, 1 out]
              }
              frame Disabled {
              }
            }
          }
          frame True {
            n102 = local read "Sampling information"() -> (w197:cluster{"Fs":dbl, "#s":dbl}[])
            n103 = Index Array(array=w197) -> (element=w196:cluster{"Fs":dbl, "#s":dbl})  [unwired: 1 in]
            n104 = call "Patrick-multichannel-Sim-Aq.vi"("Data"=w193, "sampling info"=w196) -> ("Data"=w195:waveform(dbl)[])  [unwired: 5 in]
          }
        }
        "Backlog" <- w126
        n105 = call "decimate_waveforms.vi"("decimating factor"="decimating factor", "averaging"=FALSE, "Input Signal"=w132) -> ("Decimated Waveforms"=w131:waveform(dbl)[])  [unwired: 7 in, 1 out]
        n106 = case shown="True" "measure offset" {
          tunnel: w131 -> [_ w198]
          frame False {
          }
          frame True {
            n107 = for {
              tunnel: [w202] -> w199 mode=indexing
              tunnel: w198 -> [w201] mode=indexing
              n108 = Unbundle By Name(w201) -> ("Y"=w200:dbl[])
              n109 = call-poly <vilib>:"Mean.vi"("X"=w200) -> ("mean"=w202:dbl)  [unwired: 1 out]
            }
            "offsets" <- w199
          }
        }
        n110 = for {
          tunnel: w131 -> [w205] mode=indexing
          tunnel: [w204] -> w124 mode=indexing
          tunnel: w140 -> [w203] mode=indexing
          n111 = Subtract(x=w205, y=w203) -> (x-y=w204:waveform(dbl))
        }
        "Waveform Graph" <- w124
        n112 = for {
          tunnel: w124 -> [w208] mode=indexing
          tunnel: [w207] -> w125 mode=indexing
          tunnel: "Gain" -> [w206] mode=indexing
          n113 = Divide(x=w208, y=w206) -> (x/y=w207:waveform(dbl))
        }
        n114 = case shown="False" w128 {
          tunnel: w136 -> [w172 _]
          tunnel: w127 -> [w163 _]
          frame False {
            n115 = Index Array(array=w172) -> (element #1=w171:refnum<k21>, element #2=w170:refnum<k21>, element #3=w169:refnum<k21>, element #4=w168:refnum<k21>)  [unwired: 4 in]
            n116 = Index Array(array=w163) -> (element #1=w167:waveform(dbl)[], element #2=w166:waveform(dbl)[], element #3=w165:waveform(dbl)[], element #4=w164:waveform(dbl)[])  [unwired: 8 in]
            n117 = disable-structure shown="Enabled" {
              disable-tunnel: w171 -> [w180 _]
              disable-tunnel: w170 -> [w179 _]
              disable-tunnel: w169 -> [w178 _]
              disable-tunnel: w168 -> [w177 _]
              disable-tunnel: w167 -> [w176 _]
              disable-tunnel: w166 -> [w175 _]
              disable-tunnel: w165 -> [w174 _]
              disable-tunnel: w164 -> [w173 _]
              frame Enabled {
                n118 = call-poly <vilib>:"DAQmx Write.vi"("task/channels in"=w180, "data"=w176) -> ()  [unwired: 11 in, 3 out]
                n119 = call-poly <vilib>:"DAQmx Write.vi"("task/channels in"=w179, "data"=w175) -> ()  [unwired: 11 in, 3 out]
                n120 = call-poly <vilib>:"DAQmx Write.vi"("task/channels in"=w178, "data"=w174) -> ()  [unwired: 11 in, 3 out]
                n121 = call-poly <vilib>:"DAQmx Write.vi"("task/channels in"=w177, "data"=w173) -> ()  [unwired: 11 in, 3 out]
              }
              frame Disabled {
              }
            }
          }
          frame True {
          }
        }
        n122 = call "Output FGV.vi"("Function"=enum16{"write", "read"}."write", "Output"=w127) -> ()  [unwired: 4 in, 2 out]
        n123 = call "Input Signals Waveform FGV.vi"("Function"=enum16{"write", "read"}."write", "input signal"=w125) -> ()  [unwired: 4 in, 2 out]
      }
      frame 3 {
        # "get DC"
        # "MULTIPLY &\nMULTIPLY x2"
        # "GENERATE UNITY REF\n(SINE & COSINE)"
        # "make only one reference"
        # "OR statement goes here:\nlook for changes to OSC"
        # "The code to the right sends the lockin analysis results to one graph in each tab, then sends the current value of the current tab to Display 1 and Display 2"
        # "This code does lockin analysis of the data that was read, and then displays the results.  The result is multiplied by the gain for each element of the results."
        n124 = local read "Sampling information"() -> (w287:cluster{"Fs":dbl, "#s":dbl}[])
        n125 = local read "decimating factor"() -> (w286:i32)
        n126 = Index Array(array=w287) -> (element=w296:cluster{"Fs":dbl, "#s":dbl})  [unwired: 1 in]
        n127 = local read "Remote"() -> (w310:bool)
        n128 = case shown="True" w310 {
          tunnel: [w353 w354] -> _
          frame False {
            n129 = local read "OSC Configuration"() -> (w353:T4)
          }
          frame True {
            n130 = call "OSC Configuration FGV.vi"("Function"=enum16{"write", "read"}."read") -> ("OSC Configuration"=w354:T4)  [unwired: 5 in, 1 out]
          }
        }
        n131 = Unbundle By Name(w296) -> ("Fs"=w292:dbl, "#s"=w295:dbl)
        n132 = Divide(x=w292, y=w286) -> (x/y=w268:dbl)
        n133 = Divide(x=w295, y=w286) -> (x/y=w294:dbl)
        n134 = Bundle By Name(cluster=w296, "Fs"=w268, "#s"=w294) -> (w285:cluster{"Fs":dbl, "#s":dbl})
        n135 = for {
          tunnel: w285 -> [w341]
          tunnel: w284 -> [w345]
          tunnel: [w344] -> w293 mode=indexing
          tunnel: dbl[] [0.0, 90.0] -> [w343] mode=indexing
          n136 = call <vilib>:"Sine Waveform.vi"("sampling info"=w341, "reset signal"=TRUE, "phase"=w343, "amplitude"=1.0, "frequency"=w345) -> ("signal out"=w344:waveform(dbl))  [unwired: 5 in, 1 out]
        }
        n137 = Index Array(array=w257) -> (element=w260:waveform(dbl))  [unwired: 1 in]
        n138 = for {
          tunnel: [w338] -> w261 mode=concatenating
          tunnel: w257 -> [w340]
          tunnel: w293 -> [w339] mode=indexing
          n139 = Multiply(1:w340, 2:w339) -> (0:w338:waveform(dbl)[])  [unwired: 1 in, 1 out]
        }
        n140 = Unbundle By Name(w260) -> ("t0"=w259:timestamp)
        n141 = Multiply(x="TC (s)", y=6.283185307179586) -> (x*y=w270:dbl)
        n142 = Multiply(x=w261, y=2.0) -> (x*y=w262:waveform(dbl)[])
        n143 = Reciprocal(x=w270) -> (1/x=w265:dbl)
        "filter fC (Hz)" <- w265
        n144 = for {
          tunnel: [w322] -> w263 mode=indexing
          tunnel: w262 -> [w321] mode=indexing
          tunnel: w259 -> [w320]
          n145 = Bundle By Name(cluster=w321, "t0"=w320) -> (w322:waveform(dbl))
        }
        n146 = Bundle By Name(cluster=T10 {"Topology"=enum."Butterworth", "Type"=enum."Lowpass", "Order"=1, "Lower Fc"=100.0, "Upper Fc"=200.0, "PB Ripple"=1.0, "SB Attenuation"=60.0} ("IIR filter specifications"), "Lower Fc"=w265) -> (w264:T10)
        n147 = case shown="True" "pt by pt?" {
          tunnel: [w325 w331] -> w271
          tunnel: w263 -> [w326 w330]
          tunnel: w265 -> [_ w329]
          tunnel: w268 -> [_ w328]
          tunnel: w264 -> [w324 _]
          frame False {
            n148 = call-poly <vilib>:"Digital IIR Filter.vi"("IIR filter specifications"=w324, "reset filters"=FALSE, "signal(s) in"=w326) -> ("signal(s) out"=w325:waveform(dbl)[])  [unwired: 6 in, 2 out]
          }
          frame True {
            n149 = call "Waveform N channels LP pt by pt.vi"("order"="order", "fl"=w329, "fs"=w328, "Array in"=w330) -> ("Array out"=w331:waveform(dbl)[])  [unwired: 7 in]
          }
        }
        n150 = local read "Input Signals"() -> (w283:i16)
        n151 = Decrement(x=w283) -> (x-1=w281:i16)
        n152 = Add(x=w281, y=i16 8) -> (x+y=w280:i16)
        n153 = Index Array(array=w257, index=w281) -> (element=w274:waveform(dbl))
        n154 = Index Array(array=w263, index #1=w281, index #2=w280) -> (element #1=w277:waveform(dbl), element #2=w279:waveform(dbl))
        n155 = Index Array(array=w271, index #1=w281, index #2=w280) -> (element #1=w278:waveform(dbl), element #2=w276:waveform(dbl))
        n156 = call-poly <vilib>:"Basic Averaged DC-RMS.vi"("averaging type"=enum16{"Linear", "Exponential"}."Exponential", "signals in"=w271) -> ("DC values"=w273:dbl[])  [unwired: 6 in, 3 out]
        n157 = global read "Lock-in Globles Multiple Inputs and Outputs used with FGV.vi" "Stop Lockin"() -> (w316:bool)
        n158 = Build Array(w274, w277, w276) -> (w275:waveform(dbl)[])
        n159 = Split 1D Array(array=w273, index=8) -> (first subarray=w291:dbl[], second subarray=w290:dbl[])
        n160 = for {
          tunnel: w291 -> [w332] mode=indexing
          tunnel: w290 -> [w334] mode=indexing
          tunnel: [w333] -> w258 mode=indexing
          n161 = Re/Im To Polar(2:w334, 3:w332) -> (0:w337:dbl, 1:w335:dbl)
          n162 = expression code="x * 180/pi"(w337) -> (w336:dbl)
          n163 = Build Array(w332, w334, w335, w336) -> (w333:dbl[])
        }
        "Results (X, Y, R, Theta)" <- w258
        n164 = case shown="\"FFT\"" "Tab Control" {
          tunnel: w275 -> [_ w348]
          frame "Input signals", Default {
          }
          frame "FFT" {
            n165 = global read "Lock-in Globles Multiple Inputs and Outputs used with FGV.vi" "Reset Lockin"() -> (w352:bool)
            n166 = call-poly <vilib>:"FFT Power Spectrum and PSD.vi"("averaging parameters"="averaging parameters", "restart averaging (F)"=w352, "dB On (F)"="dB On (F)", "window"="window", "time signals"=w348) -> ("Power Spectrum / PSD"=→"Waveform Graph 2":cluster{"f0":dbl, "df":dbl, "magnitude":dbl[]}[])  [unwired: 3 in, 3 out]
          }
        }
        n167 = global read "Lock-in Globles Multiple Inputs and Outputs used with FGV.vi" "Reset Lockin"() -> (w305:bool)
        n168 = Or(x=w316, y="stop") -> (x .or. y?=w314:bool)
        n169 = local read "Measure?"() -> (w300:u16[])
        n170 = Select(t=4.0 ("f"), s=w314, f=2.0) -> (s? t:f=w313:dbl)
        n171 = Decrement(x="Input Signals") -> (x-1=w307:i16)
        n172 = call "Display.vi"("Results"=w258, "Display"="Display", "Lock-in #"=w307, "Amplifier Settings"=w300) -> ("Display 1"=→"Display 1":string, "Display 2"=→"Display 2":string, "Array"=→"Display X (or R) A":dbl[], "Array 2"=→"Display Y (or Theta) A":dbl[])  [unwired: 3 in]
        n173 = Build Array(w274, w277, w279, w278, w276) -> ()  [unwired: 1 out]
        n174 = Select(t=5.0, s=w305, f=w313) -> (s? t:f=w311:dbl)
        n175 = call "Results FGV.vi"("Function"=enum16{"write", "read"}."write", "Input Signals"=w258) -> ()  [unwired: 4 in, 2 out]
      }
      frame 4 {
        # "This code stops the AI/AO Tasks, erases them, and ends program execution."
        n176 = local read "simulate?"() -> (w356:bool)
        n177 = case shown="False" w356 {
          frame False {
            n178 = disable-structure shown="Enabled" {
              frame Enabled {
                n179 = local read "AO Task"() -> (w362:refnum<k21>[])
                n180 = local read "AI task"() -> (w363:refnum<k21>[])
                n181 = flat-sequence {
                  tunnel: w363 -> [w376]
                  tunnel: [w375] -> w366
                  tunnel: w362 -> [w375]
                  tunnel: [w374] -> w365
                  tunnel: w366 -> [w382]
                  tunnel: w365 -> [w381]
                  tunnel: [w381] -> w361
                  tunnel: [w380] -> w360
                  frame #0 {
                    n182 = for {
                      tunnel: w376 -> [w379] mode=indexing
                      tunnel: [w377] -> w374 mode=indexing
                      n183 = Wait (ms)(milliseconds to wait=u32 50) -> ()  [unwired: 1 out]
                      n184 = call <vilib>:"DAQmx Stop Task.vi"("task/channels in"=w379) -> ("task out"=w377:refnum<k21>)  [unwired: 13 in, 1 out]
                    }
                  }
                  frame #1 {
                    n185 = for {
                      tunnel: w382 -> [w385] mode=indexing
                      tunnel: [w383] -> w380 mode=indexing
                      n186 = Wait (ms)(milliseconds to wait=u32 50) -> ()  [unwired: 1 out]
                      n187 = call <vilib>:"DAQmx Stop Task.vi"("task/channels in"=w385) -> ("task out"=w383:refnum<k21>)  [unwired: 13 in, 1 out]
                    }
                  }
                }
                n188 = flat-sequence {
                  tunnel: w361 -> [w368]
                  tunnel: w360 -> [w367]
                  tunnel: [w367] -> w364
                  tunnel: w364 -> [w371]
                  frame #0 {
                    n189 = for {
                      tunnel: w368 -> [w370] mode=indexing
                      n190 = call <vilib>:"DAQmx Clear Task.vi"("task in"=w370) -> ()  [unwired: 14 in, 1 out]
                      n191 = Wait (ms)(milliseconds to wait=u32 50) -> ()  [unwired: 1 out]
                    }
                  }
                  frame #1 {
                    n192 = for {
                      tunnel: w371 -> [w373] mode=indexing
                      n193 = call <vilib>:"DAQmx Clear Task.vi"("task in"=w373) -> ()  [unwired: 14 in, 1 out]
                      n194 = Wait (ms)(milliseconds to wait=u32 50) -> ()  [unwired: 1 out]
                    }
                  }
                }
              }
              frame Disabled {
              }
            }
          }
          frame True {
          }
        }
      }
      frame 5 {
        # "This code stops AI/AO tasks, deletes them, and restarts program execution."
        n195 = local read "simulate?"() -> (w386:bool)
        n196 = case shown="False" w386 {
          frame False {
            n197 = disable-structure shown="Enabled" {
              frame Enabled {
                n198 = local read "AO Task"() -> (w390:refnum<k21>[])
                n199 = local read "AI task"() -> (w391:refnum<k21>[])
                n200 = flat-sequence {
                  tunnel: w391 -> [w399]
                  tunnel: [w398] -> w396
                  tunnel: w390 -> [w398]
                  tunnel: [w397] -> w395
                  tunnel: w396 -> [w405]
                  tunnel: w395 -> [w404]
                  tunnel: [w404] -> w394
                  tunnel: [w403] -> w393
                  tunnel: w394 -> [w409]
                  tunnel: w393 -> [w410]
                  tunnel: [w410] -> w392
                  tunnel: w392 -> [w413]
                  frame #0 {
                    n201 = for {
                      tunnel: w399 -> [w402] mode=indexing
                      tunnel: [w400] -> w397 mode=indexing
                      n202 = Wait (ms)(milliseconds to wait=u32 50) -> ()  [unwired: 1 out]
                      n203 = call <vilib>:"DAQmx Stop Task.vi"("task/channels in"=w402) -> ("task out"=w400:refnum<k21>)  [unwired: 13 in, 1 out]
                    }
                  }
                  frame #1 {
                    n204 = for {
                      tunnel: w405 -> [w408] mode=indexing
                      tunnel: [w406] -> w403 mode=indexing
                      n205 = Wait (ms)(milliseconds to wait=u32 50) -> ()  [unwired: 1 out]
                      n206 = call <vilib>:"DAQmx Stop Task.vi"("task/channels in"=w408) -> ("task out"=w406:refnum<k21>)  [unwired: 13 in, 1 out]
                    }
                  }
                  frame #2 {
                    n207 = for {
                      tunnel: w409 -> [w412] mode=indexing
                      n208 = call <vilib>:"DAQmx Clear Task.vi"("task in"=w412) -> ()  [unwired: 14 in, 1 out]
                      n209 = Wait (ms)(milliseconds to wait=u32 50) -> ()  [unwired: 1 out]
                    }
                  }
                  frame #3 {
                    n210 = for {
                      tunnel: w413 -> [w415] mode=indexing
                      n211 = call <vilib>:"DAQmx Clear Task.vi"("task in"=w415) -> ()  [unwired: 14 in, 1 out]
                      n212 = Wait (ms)(milliseconds to wait=u32 50) -> ()  [unwired: 1 out]
                    }
                  }
                }
              }
              frame Disabled {
              }
            }
          }
          frame True {
          }
        }
      }
    }
  }
